vi "Discard Non-Analog Channels.vi"(7 "Channels In (-)":i32[](array[numeric])=[31, 31, 31, 31, 31, 31, 31, 31, 31, 31, 31, 31, 31, 31, 31, 31], 9 "Ranges In":string[](array[string]), 10 "Channels In":i32[](array[numeric])) -> (1 "Ranges Out":string[](array[string]), 2 "Channels Out":i32[](array[numeric]), 4 "FIO/EIO Analog Enable":i32, 5 "Channels Out (-)":i32[](array[numeric]))   [LabVIEW 2020]
panel:
  # "This is a simply VI to remove non-analog channels from the channels/ranges arrays.  The output\narrays contain analog channels only and can then be used to configure ranges.  Also calculates\nthe value to pass to enable the needed analog channels on the U3."
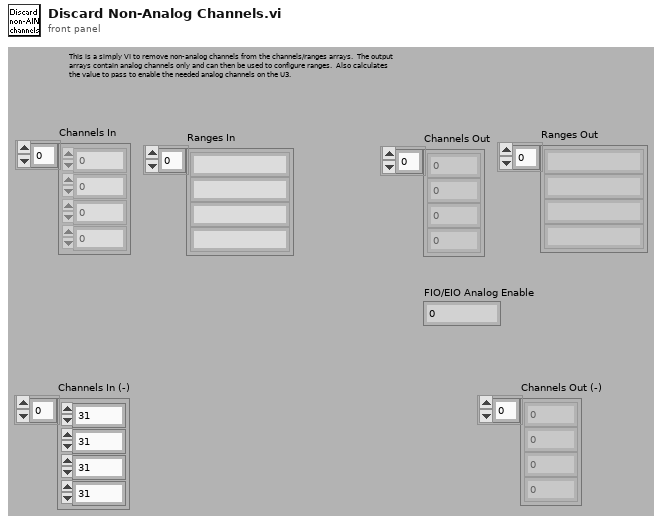
[diagram p1: front panel]
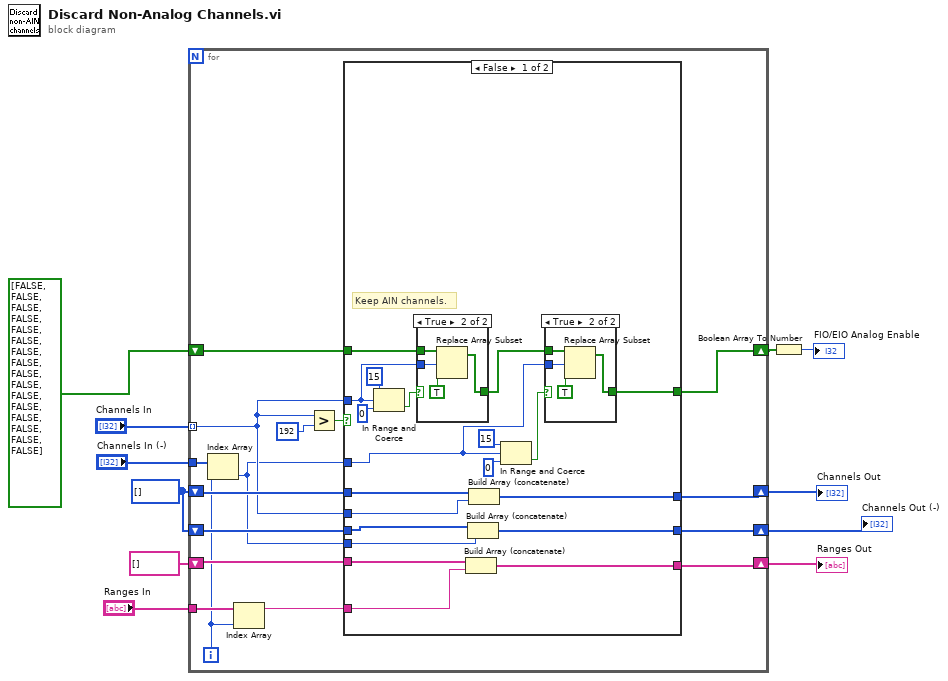
[diagram p0: block diagram]
diagram:
  w3 = i32[] []
  n1 = for {
    shift-right: [w25] -> w8
    shift-left: w3 -> [w26]
    shift-right: [w22] -> w7
    shift-left: string[] [] -> [w23]
    tunnel: "Channels In" -> [w21] mode=indexing
    tunnel: "Ranges In" -> [w18]
    shift-right: [w19] -> w5
    shift-left: bool[] [FALSE, FALSE, FALSE, FALSE, FALSE, FALSE, FALSE, FALSE, FALSE, FALSE, FALSE, FALSE, FALSE, FALSE, FALSE, FALSE] -> [w20]
    shift-right: [w16] -> w1
    shift-left: w3 -> [w15]
    tunnel: "Channels In (-)" -> [w14]
    i -> [w13]
    n2 = Index Array(array=w14, index=w13) -> (element=w12:i32)
    n3 = Index Array(array=w18, index=w13) -> (element=w17:string)
    n4 = Greater?(x=w21, y=192) -> (0:w27:bool)
    n5 = case shown="False" w27 {
      tunnel: w21 -> [w46 _]
      tunnel: w26 -> [w47 w61]
      tunnel: [w45 w61] -> w25
      tunnel: w23 -> [w44 w60]
      tunnel: w17 -> [w43 _]
      tunnel: [w42 w60] -> w22
      tunnel: w21 -> [w37 _]
      tunnel: w20 -> [w38 w59]
      tunnel: [w28 w59] -> w19
      tunnel: [w36 w58] -> w16
      tunnel: w15 -> [w34 w58]
      tunnel: w12 -> [w35 _]
      tunnel: w12 -> [w29 _]
      frame False {
        # "Keep AIN channels."
        n6 = In Range and Coerce(upper limit=15, x=w37, lower limit=0) -> (In Range?=w41:bool)  [unwired: 1 out]
        n7 = case shown="True" w41 {
          tunnel: w38 -> [w53 w56]
          tunnel: [w53 w54] -> w32
          tunnel: w37 -> [_ w57]
          frame False {
          }
          frame True {
            n8 = Replace Array Subset(array=w56, new element=TRUE, index=w57) -> (w54:bool[])
          }
        }
        n9 = Build Array (concatenate)(w44, w43) -> (w42:string[])
        n10 = Build Array (concatenate)(w34, w35) -> (w36:i32[])
        n11 = Build Array (concatenate)(w47, w46) -> (w45:i32[])
        n12 = In Range and Coerce(upper limit=15, x=w29, lower limit=0) -> (In Range?=w33:bool)  [unwired: 1 out]
        n13 = case shown="True" w33 {
          tunnel: w32 -> [w48 w51]
          tunnel: [w48 w49] -> w28
          tunnel: w29 -> [_ w52]
          frame False {
          }
          frame True {
            n14 = Replace Array Subset(array=w51, new element=TRUE, index=w52) -> (w49:bool[])
          }
        }
      }
      frame True {
      }
    }
  }
  "Channels Out" <- w8
  "Ranges Out" <- w7
  "Channels Out (-)" <- w1
  n15 = Boolean Array To Number(Boolean array=w5) -> (number=→"FIO/EIO Analog Enable":u32)
